vi "ReadConfig.vi"(8 "error in (no error)":errorcluster, 11 "SensorBase in":refnum<class "SensorBase.lvclass">) -> (0 "error out":errorcluster, 2 "Config":variant, 3 "SensorBase out":refnum<class "SensorBase.lvclass">)   [LabVIEW 2014, in "SensorPlugins.lvlib" / "SensorBase.lvclass"]
uses:
  SensorBase.lvclass
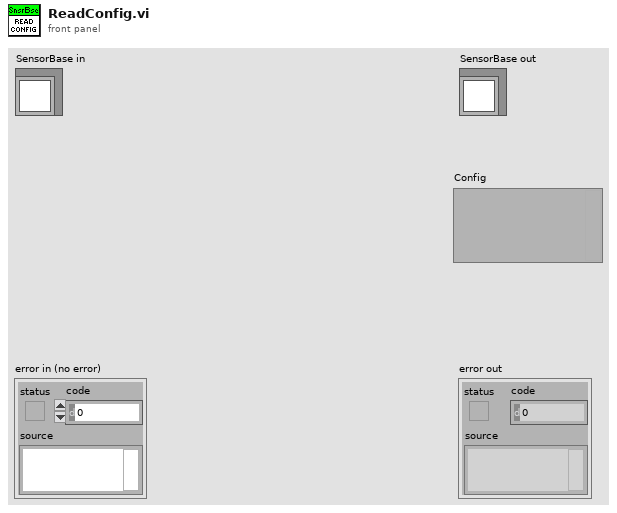
[diagram p1: front panel]
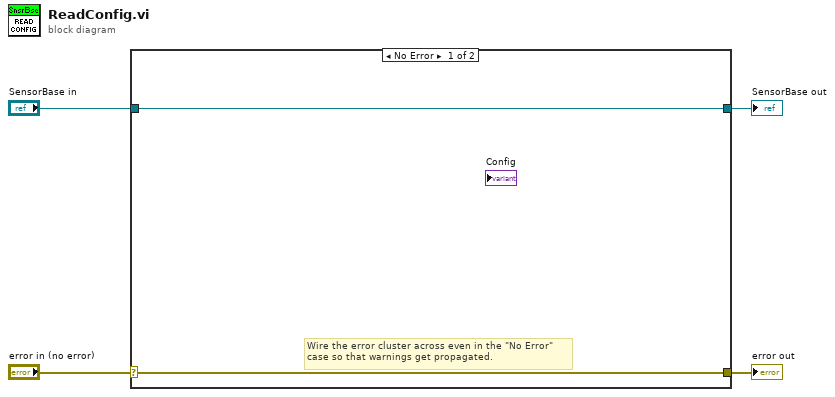
[diagram p0: block diagram]
diagram:
  n1 = case shown="No Error" "error in (no error)" {
    selector: "error in (no error)" -> [w5 w8]
    tunnel: [w5 w8] -> w3
    tunnel: [w6 w7] -> w1
    tunnel: "SensorBase in" -> [w6 w7]
    frame No Error {
      # "Wire the error cluster across even in the \"No Error\"\ncase so that warnings get propagated."
    }
    frame Error {
    }
  }
  "error out" <- w3
  "SensorBase out" <- w1
